vi "Classify.vi"(8 "error in (no error)":errorcluster, 10 "msg to Log":string, 11 "Log in":refnum<class "Log.lvclass">) -> (0 "error out":errorcluster, 3 "Log out":refnum<class "Log.lvclass">)   [LabVIEW 2018, in "Log.lvclass"]
uses:
  Log.lvclass
  Log.lvclass/Log.ctl
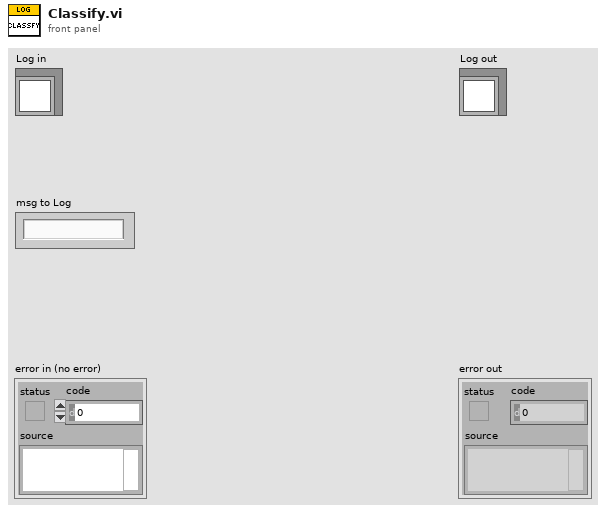
[diagram p1: front panel]
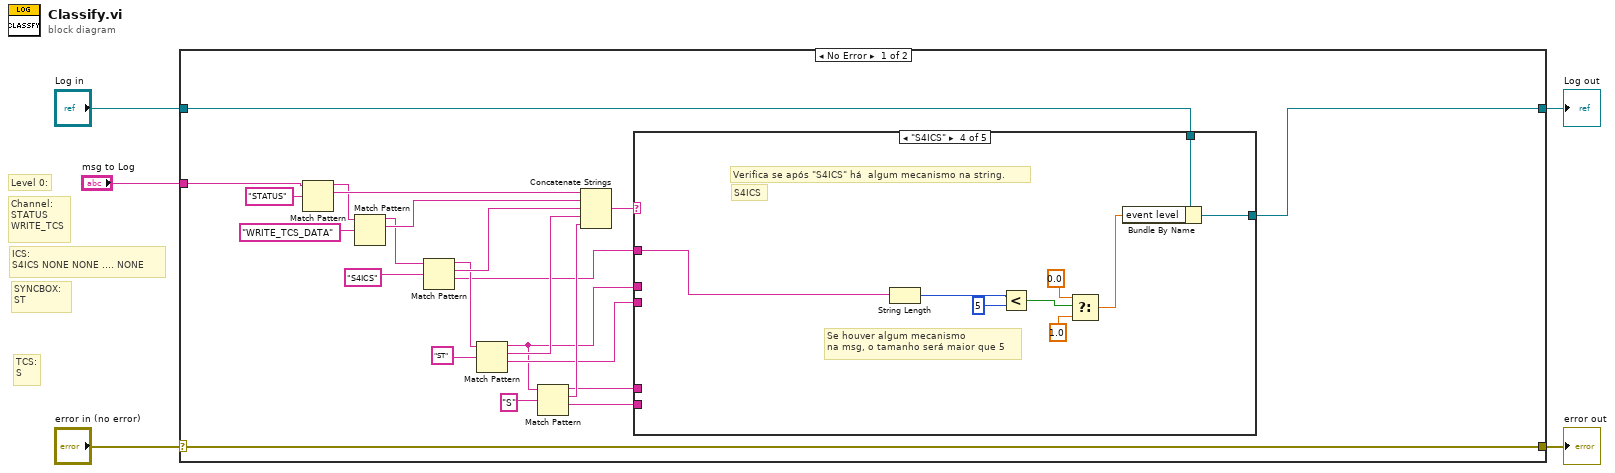
[diagram p0: block diagram]
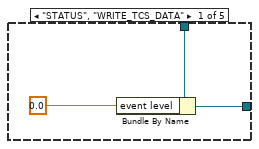
[diagram p2: hidden frame]
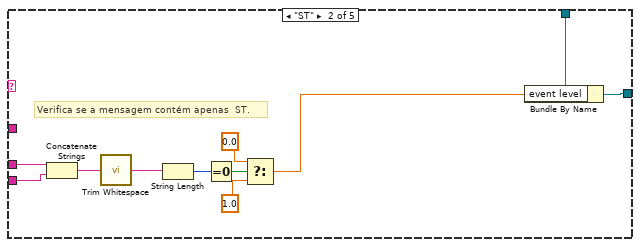
[diagram p3: hidden frame]
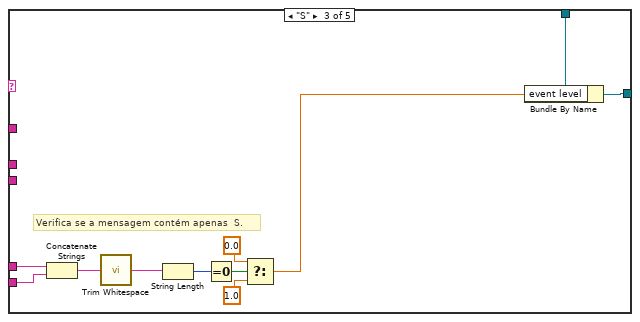
[diagram p4: hidden frame]
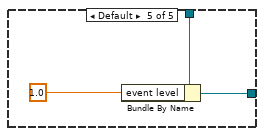
[diagram p5: hidden frame]
diagram:
  # "TCS:\nS"
  # "SYNCBOX:\nST"
  # "Level 0:"
  # "ICS:\nS4ICS NONE NONE .... NONE"
  # "Channel:\nSTATUS\nWRITE_TCS"
  n1 = case shown="No Error" "error in (no error)" {
    selector: "error in (no error)" -> [w28 w67]
    tunnel: [w28 w67] -> w4
    tunnel: [w19 w66] -> w2
    tunnel: "Log in" -> [w20 w66]
    tunnel: "msg to Log" -> [w26 _]
    frame No Error {
      n2 = Match Pattern(string=w26, regular expression="STATUS") -> (before substring=w17:string, match substring=w25:string)  [unwired: 1 in, 2 out]
      n3 = Match Pattern(string=w17, regular expression="WRITE_TCS_DATA") -> (before substring=w16:string, match substring=w24:string)  [unwired: 1 in, 2 out]
      n4 = Match Pattern(string=w16, regular expression="S4ICS") -> (before substring=w15:string, match substring=w23:string, after substring=w12:string)  [unwired: 1 in, 1 out]
      n5 = Match Pattern(string=w15, regular expression="ST") -> (before substring=w8:string, match substring=w22:string, after substring=w9:string)  [unwired: 1 in, 1 out]
      n6 = Match Pattern(string=w8, regular expression="S") -> (before substring=w7:string, match substring=w18:string, after substring=w6:string)  [unwired: 1 in, 1 out]
      n7 = Concatenate Strings(w25, w24, w23, w22, w18) -> (w21:string)
      n8 = case shown="\"S4ICS\"" w21 {
        tunnel: w20 -> [w31 w34 w47 w60 w65]
        tunnel: [w29 w33 w46 w58 w64] -> w19
        tunnel: w12 -> [_ _ _ w57 _]
        tunnel: w8 -> [_ w42 _ _ _]
        tunnel: w9 -> [_ w41 _ _ _]
        tunnel: w7 -> [_ _ w44 _ _]
        tunnel: w6 -> [_ _ w43 _ _]
        frame "STATUS", "WRITE_TCS_DATA" {
          n9 = Bundle By Name(cluster=w31, "event level"=0.0 ("current level")) -> (w29:refnum<class "Log.lvclass">)
        }
        frame "ST" {
          # "Verifica se a mensagem contém apenas  ST."
          n10 = Concatenate Strings(w42, w41) -> (w40:string)
          n11 = call <vilib>:"Trim Whitespace.vi"("string"=w40) -> ("trimmed string"=w39:string)  [unwired: 1 in]
          n12 = String Length(string=w39) -> (length=w38:i32)
          n13 = Equal To 0?(x=w38) -> (x = 0?=w37:bool)
          n14 = Select(t=0.0, s=w37, f=1.0) -> (s? t:f=w32:dbl)
          n15 = Bundle By Name(cluster=w34, "event level"=w32) -> (w33:refnum<class "Log.lvclass">)
        }
        frame "S" {
          # "Verifica se a mensagem contém apenas  S."
          n16 = Concatenate Strings(w44, w43) -> (w53:string)
          n17 = call <vilib>:"Trim Whitespace.vi"("string"=w53) -> ("trimmed string"=w52:string)  [unwired: 1 in]
          n18 = String Length(string=w52) -> (length=w51:i32)
          n19 = Equal To 0?(x=w51) -> (x = 0?=w50:bool)
          n20 = Select(t=0.0, s=w50, f=1.0) -> (s? t:f=w45:dbl)
          n21 = Bundle By Name(cluster=w47, "event level"=w45) -> (w46:refnum<class "Log.lvclass">)
        }
        frame "S4ICS" {
          # "Se houver algum mecanismo\nna msg, o tamanho será maior que 5"
          # "Verifica se após \"S4ICS\" há  algum mecanismo na string."
          # "S4ICS"
          n22 = String Length(string=w57) -> (length=w56:i32)
          n23 = Less?(x=w56, y=5) -> (x < y?=w54:bool)
          n24 = Select(t=0.0, s=w54, f=1.0) -> (s? t:f=w59:dbl)
          n25 = Bundle By Name(cluster=w60, "event level"=w59) -> (w58:refnum<class "Log.lvclass">)
        }
        frame Default {
          n26 = Bundle By Name(cluster=w65, "event level"=1.0) -> (w64:refnum<class "Log.lvclass">)
        }
      }
    }
    frame Error {
    }
  }
  "error out" <- w4
  "Log out" <- w2
